vi "MoAgSy_GPG.appenddata2Variant.vi"(2 "initData":variant) -> (16 "dup initData":variant)   [LabVIEW 2009, in "MoAgSy.lvlib" / "MoAgSy_GPG.lvclass"]
uses:
  MoAgSy_GPG.lvclass
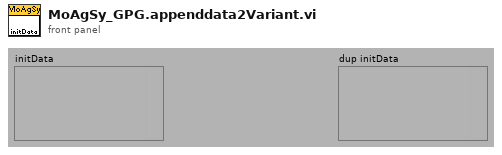
[diagram p1: front panel]
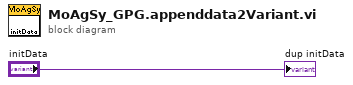
[diagram p0: block diagram]
diagram:
  "dup initData" <- "initData"
